vi "Cluster To Array 2012 NIVerified.vi"(11 "Cluster":T1={"String"="I am a string", "Boolean"=TRUE, "Numeric"=17.0, "Array - String"=[]}) -> ()   [LabVIEW 2012]
doc: "The attached Cluster To Array.vi example shows a method for handling each element of a cluster individually as an alternative to the Unbundle or Unbundle By Name functions. Unbundling very large clusters with many different data types can create complicated and visually challenging LabVIEW Block Diagrams with many wires. This fexample provides an alternative that is cleaner and takes up less space on the Block Diagram.\nIn the example, the cluster is converted to an array of controls via a property node. The values of each cluster element are then extracted individually in Variant form with an auto-indexing For Loop. The Get TypeInfoVI is then used to determine the LabVIEW Data Type of each element. (The GetTypeInfo and other VIs relating to Variants are located here: Program Files\\National Instruments\\LabVIEW 2011\\vi.lib\\Utility\\VariantDataType) Finally, a case structure and the Variant To Data function are used to handle each element differently based on its LabVIEW Data Type. In the case of the attached example, String, Boolean, Double Float, and Array data are each displayed as their distinct data type."
uses:
  <vilib>/Utility/VariantDataType/VariantType.lvlib
panel:
  out "data":string[](array[string])
  out "Numeric":dbl
  out "String":string
  out "Boolean":bool
  # "Overview: This VI shows a method for handling each element of a cluster individually as an\nalternative to the Unbundle or Unbundle By Name functions.\nRequirements: LabVIEW 2012 (or compatible).\nInstructions:\n1. Input data to the Cluster.\n2. Run the VI."
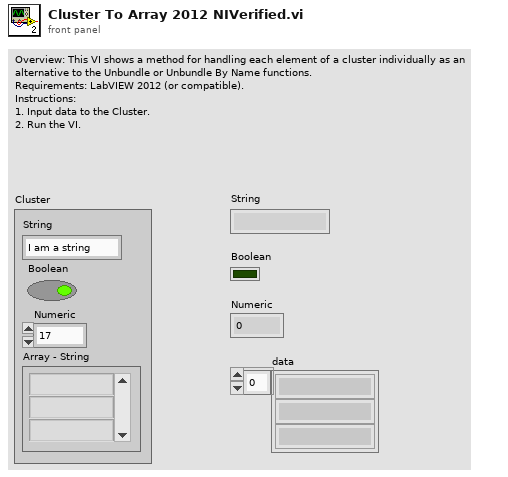
[diagram p1: front panel]
types:
  T1 = cluster{"String":string, "Boolean":bool, "Numeric":dbl, "Array - String":string[]}
  T2 = typedef "VariantType.lvlib/Type.ctl" = enum8{"Invalid Type", "Void", "I8", "I16", "I32", "I64", "U8", "U16", "U32", "U64", "Single Float", "Double Float", "Extended Float", "Single Complex", "Double Complex", "Extended Complex", "Enum U8", "Enum U16", "Enum U32", "Enum U64", "Single Float With Unit", "Double Float With Unit", "Extended Float With Unit", "Single Complex with Unit", "Double Complex with Unit", "Extended Complex with Unit", "Boolean", "String", "Path", "Picture", "Tag", "Array", "Cluster", "Variant", "LV Variant", "Waveform", "Timestamp", "Digital Waveform", "Digital Data", "ExpressData", "Refnum", "External Data", "VI", "Poly VI", "LabVIEW Class Instance", "Fixed Point"}
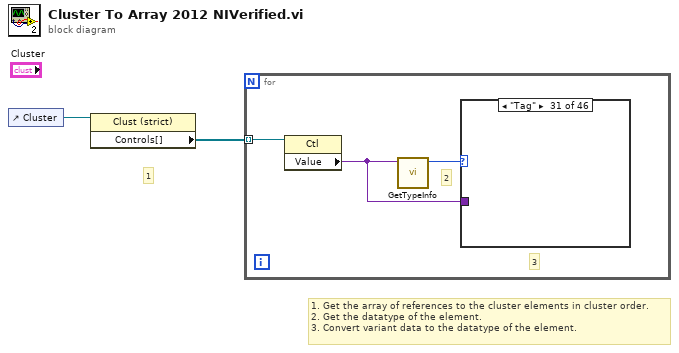
[diagram p0: block diagram]
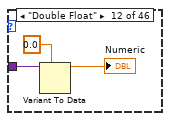
[diagram p13: hidden frame]
diagram:
  # "1. Get the array of references to the cluster elements in cluster order.\n2. Get the datatype of the element.\n3. Convert variant data to the datatype of the element."
  # "1"
  n1 = control-ref of="Cluster"() -> (w2:refnum<vi>)
  n2 = property class="Clust (strict)"(reference=w2) -> ("Controls[]"=w1:refnum<vi>[])  [unwired: 1 in, 2 out]
  n3 = for {
    tunnel: w1 -> [w4] mode=indexing
    # "3"
    # "2"
    n4 = property class="Ctl"(reference=w4) -> ("Value"=w3:variant)  [unwired: 1 in, 2 out]
    n5 = call <vilib>:"GetTypeInfo.vi"("Variant"=w3) -> ("Type Enum"=w5:T2)  [unwired: 6 in, 4 out]
    n6 = case shown="\"Tag\"" w5 {
      tunnel: w3 -> [_ _ _ _ _ _ _ _ _ _ _ w8 _ _ _ _ _ _ _ _ _ _ _ _ _ _ w11 w14 _ _ _ w17 _ _ _ _ _ _ _ _ _ _ _ _ _ _]
      frame "Invalid Type", Default {
      }
      frame "Void" {
      }
      frame "I8" {
      }
      frame "I16" {
      }
      frame "I32" {
      }
      frame "I64" {
      }
      frame "U8" {
      }
      frame "U16" {
      }
      frame "U32" {
      }
      frame "U64" {
      }
      frame "Single Float" {
      }
      frame "Double Float" {
        n7 = Variant To Data(type=0.0, Variant=w8) -> (data=→"Numeric":dbl)  [unwired: 1 in, 1 out]
      }
      frame "Extended Float" {
      }
      frame "Single Complex" {
      }
      frame "Double Complex" {
      }
      frame "Extended Complex" {
      }
      frame "Enum U8" {
      }
      frame "Enum U16" {
      }
      frame "Enum U32" {
      }
      frame "Enum U64" {
      }
      frame "Single Float With Unit" {
      }
      frame "Double Float With Unit" {
      }
      frame "Extended Float With Unit" {
      }
      frame "Single Complex with Unit" {
      }
      frame "Double Complex with Unit" {
      }
      frame "Extended Complex with Unit" {
      }
      frame "Boolean" {
        n8 = Variant To Data(type=TRUE, Variant=w11) -> (data=→"Boolean":bool)  [unwired: 1 in, 1 out]
      }
      frame "String" {
        n9 = Variant To Data(type="", Variant=w14) -> (data=→"String":string)  [unwired: 1 in, 1 out]
      }
      frame "Path" {
      }
      frame "Picture" {
      }
      frame "Tag" {
      }
      frame "Array" {
        n10 = Variant To Data(type=string[] [], Variant=w17) -> (data=→"data":string[])  [unwired: 1 in, 1 out]
      }
      frame "Cluster" {
      }
      frame "Variant" {
      }
      frame "LV Variant" {
      }
      frame "Waveform" {
      }
      frame "Timestamp" {
      }
      frame "Digital Waveform" {
      }
      frame "Digital Data" {
      }
      frame "ExpressData" {
      }
      frame "Refnum" {
      }
      frame "External Data" {
      }
      frame "VI" {
      }
      frame "Poly VI" {
      }
      frame "LabVIEW Class Instance" {
      }
      frame "Fixed Point" {
      }
    }
  }
